vi "Filter Childless Top Nodes.vi"(11 "All Items":T1(array[cluster])) -> (3 "Filtered Items":T1(array[cluster]))   [LabVIEW 2020, in "Result Model.lvclass"]
uses:
  Result Model.lvclass
  Result Model.lvclass/Result Model.ctl
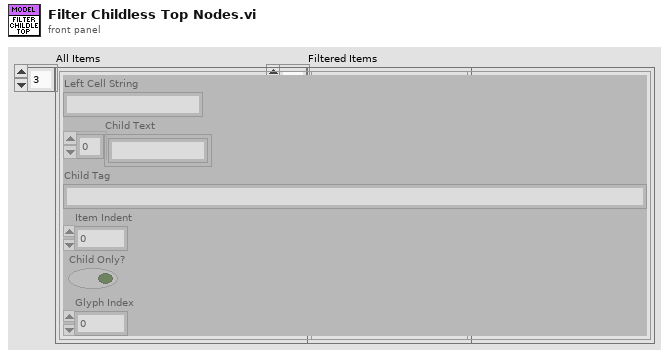
[diagram p1: front panel]
types:
  T1 = cluster{"Left Cell String":string, "Child Text":string[], "Child Tag":string, "Item Indent":i32, "Child Only?":bool, "Glyph Index":i32}[]
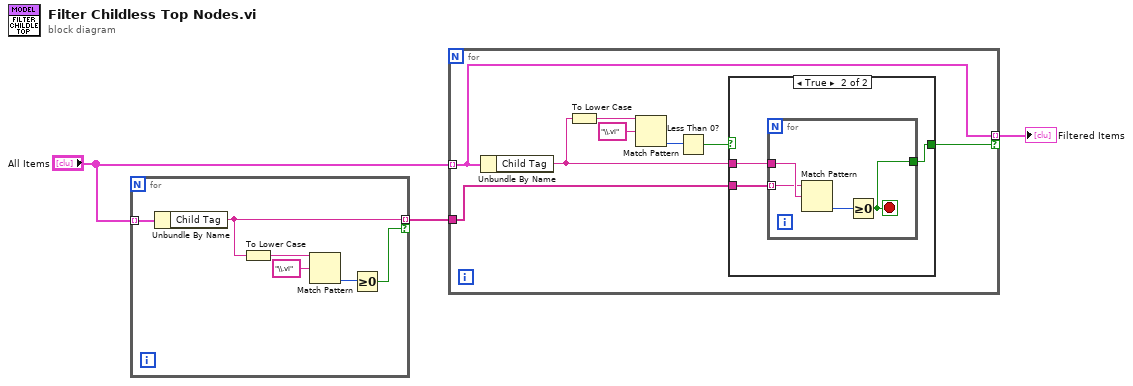
[diagram p0: block diagram]
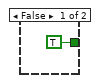
[diagram p2: hidden frame]
diagram:
  n1 = for {
    tunnel: "All Items" -> [w9] mode=indexing
    tunnel: [w4] -> w2 mode=indexing if=w5
    n2 = Unbundle By Name(w9) -> ("Child Tag"=w4:string)
    n3 = To Lower Case(string=w4) -> (all lower case string=w7:string)
    n4 = Match Pattern(string=w7, regular expression="\\.vi") -> (offset past match=w6:i32)  [unwired: 1 in, 3 out]
    n5 = Greater Or Equal To 0?(x=w6) -> (x >= 0?=w5:bool)
  }
  n6 = for {
    tunnel: "All Items" -> [w17] mode=indexing
    tunnel: [w17] -> w1 mode=indexing if=w10
    tunnel: w2 -> [w11]
    n7 = Unbundle By Name(w17) -> ("Child Tag"=w12:string)
    n8 = To Lower Case(string=w12) -> (all lower case string=w15:string)
    n9 = Match Pattern(string=w15, regular expression="\\.vi") -> (offset past match=w14:i32)  [unwired: 1 in, 3 out]
    n10 = Less Than 0?(x=w14) -> (x < 0?=w13:bool)
    n11 = case shown="True" w13 {
      tunnel: w12 -> [_ w21]
      tunnel: w11 -> [_ w20]
      tunnel: [TRUE w19] -> w10
      frame False {
      }
      frame True {
        n12 = for {
          tunnel: w21 -> [w25]
          tunnel: [w23] -> w19
          tunnel: w20 -> [w22] mode=indexing
          stop <- w23 stop-if-true
          n13 = Match Pattern(string=w22, regular expression=w25) -> (offset past match=w24:i32)  [unwired: 1 in, 3 out]
          n14 = Greater Or Equal To 0?(x=w24) -> (x >= 0?=w23:bool)
        }
      }
    }
  }
  "Filtered Items" <- w1
